vi "Verify Combinations.vi"(5 "Options":T1, 7 "Test VI (caller)":string, 8 "error in":errorcluster, 9 "map (control name -> array of variants)":map{string, variant[]}(c390), 10 "VI Refnum":refnum<vi>) -> (0 "error out":errorcluster, 1 "Failure Message":string, 2 "Passed?":bool)   [LabVIEW 2020, in "Approval Tests.lvlib"]
uses:
  Approval Tests.lvlib
  Options.ctl
  Reporter/Reporter.lvclass
  Printer/Printer.lvclass
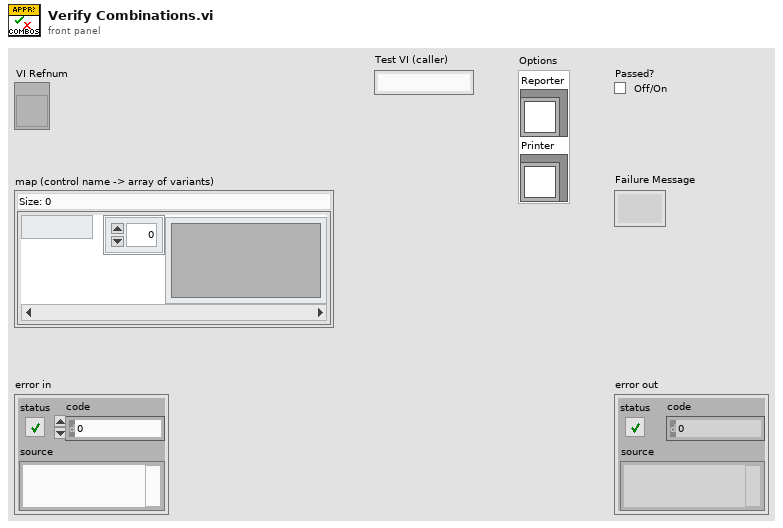
[diagram p1: front panel]
types:
  T1 = typedef "Approval Tests.lvlib/Options.ctl" = cluster{"Reporter":refnum<class "Reporter.lvclass">, "Printer":refnum<class "Printer.lvclass">}
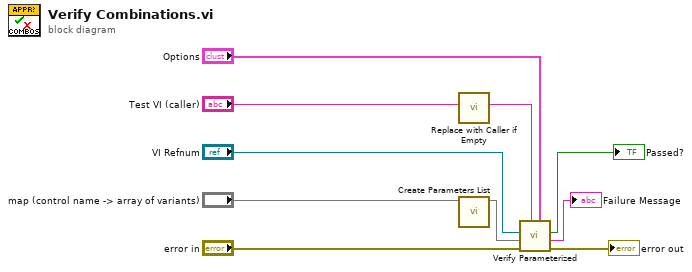
[diagram p0: block diagram]
diagram:
  n1 = call "Replace with Caller if Empty.vi"("Test VI (caller) in"="Test VI (caller)") -> ("Test VI (caller) out"=w1:string)  [unwired: 10 in]
  n2 = call "Create Parameters List.vi"("Combo map"="map (control name -> array of variants)") -> ("Set of Parameters"=w5:set{map{string, variant}})  [unwired: 10 in]
  n3 = call "Verify Parameterized.vi"("Options"="Options", "Test VI (caller)"=w1, "error in (no error)"="error in", "Set (map: control name  -> value as variant)"=w5, "VI in"="VI Refnum") -> ("error out"=→"error out":errorcluster, "Failure Message"=→"Failure Message":string, "Passed?"=→"Passed?":bool)  [unwired: 4 in]
